vi "GET Ramp Rate.vi"() -> (0 "Ramp Rate":dbl)   [LabVIEW 2013]
uses:
  Action.ctl
  Experimental Parameters FGV Selector.ctl
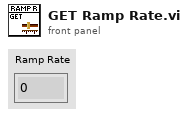
[diagram p1: front panel]
types:
  T1 = typedef "Experimental Parameters FGV Selector.ctl" = enum16{"Number of Samples", "Actuation Direction", "Ramp Rate"}
  T2 = typedef "Action.ctl" = enum16{"GET", "PUT", "DELETE"}
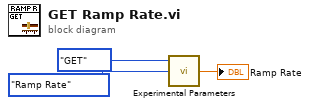
[diagram p0: block diagram]
diagram:
  n1 = call "Experimental Parameters.vi"("Experimental Parameters FGV Selector"=Experimental_Parameters_FGV_Selector."Ramp Rate", "Action"=Action."GET") -> ("Output"=→"Ramp Rate":dbl)  [unwired: 1 in]
